vi "Write Start Index.vi"(8 "error in (no error)":errorcluster, 10 "Start Index":i32, 11 "Set Delays Msg in":refnum<class "Set Delays Msg.lvclass">) -> (0 "error out":errorcluster, 3 "Set Delays Msg out":refnum<class "Set Delays Msg.lvclass">)   [LabVIEW 2021, in "BNT_ULx.lvlib" / "Set Delays Msg.lvclass"]
uses:
  Set Delays Msg.lvclass
  Set Delays Msg.lvclass/Set Delays Msg.ctl
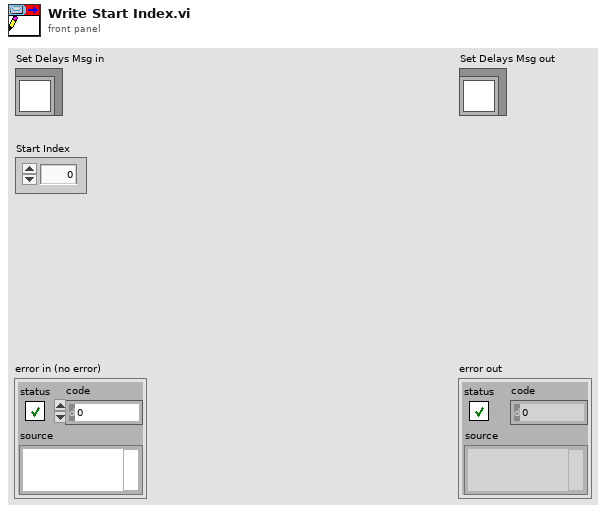
[diagram p1: front panel]
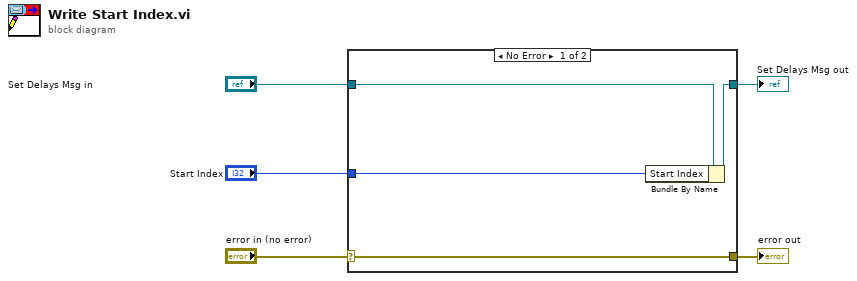
[diagram p0: block diagram]
diagram:
  n1 = case shown="No Error" "error in (no error)" {
    selector: "error in (no error)" -> [w9 w10]
    tunnel: [w9 w10] -> w4
    tunnel: [w7 w11] -> w2
    tunnel: "Set Delays Msg in" -> [w8 w11]
    tunnel: "Start Index" -> [w6 _]
    frame No Error {
      n2 = Bundle By Name(cluster=w8, "Start Index"=w6) -> (w7:refnum<class "Set Delays Msg.lvclass">)
    }
    frame Error {
    }
  }
  "error out" <- w4
  "Set Delays Msg out" <- w2
